vi "cleanup.vi"(8 "Error In":errorcluster) -> (0 "Error Out":errorcluster)   [LabVIEW 2014]
uses:
  UT FFTW States.ctl
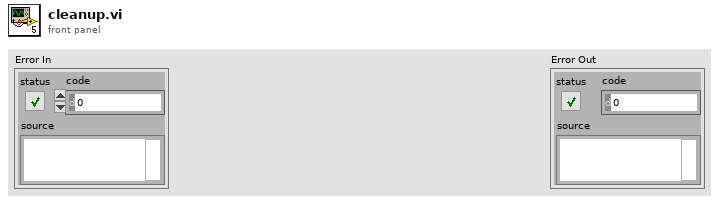
[diagram p1: front panel]
types:
  T1 = typedef "UT FFTW States.ctl" = enum16{"Init", "Transform", "Cleanup"}
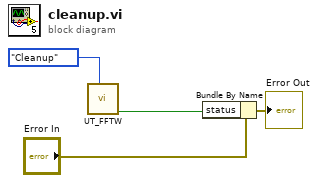
[diagram p0: block diagram]
diagram:
  n1 = call "UT_FFTW.vi"("UT FFTW States"=UT_FFTW_States."Cleanup") -> ("Error"=w1:bool)  [unwired: 9 in, 1 out]
  n2 = Bundle By Name(cluster="Error In", "status"=w1) -> (→"Error Out":errorcluster)
